vi "HEWH RLT Gather Serial Data.vi"(0 "Serial Port Ref":refnum<visa-resource-name>="COM3", 5 "GEA2 HyperData":bool, 11 "error in (no error)":errorcluster) -> (4 "Serial Data B":string[][](array[string]), 15 "error out":errorcluster)   [LabVIEW 2014]
uses:
  Support VIs/Global HEWH.vi
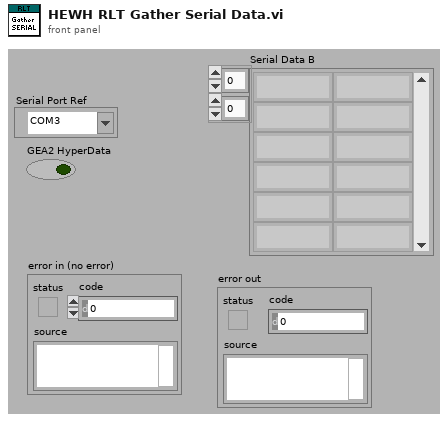
[diagram p1: front panel]
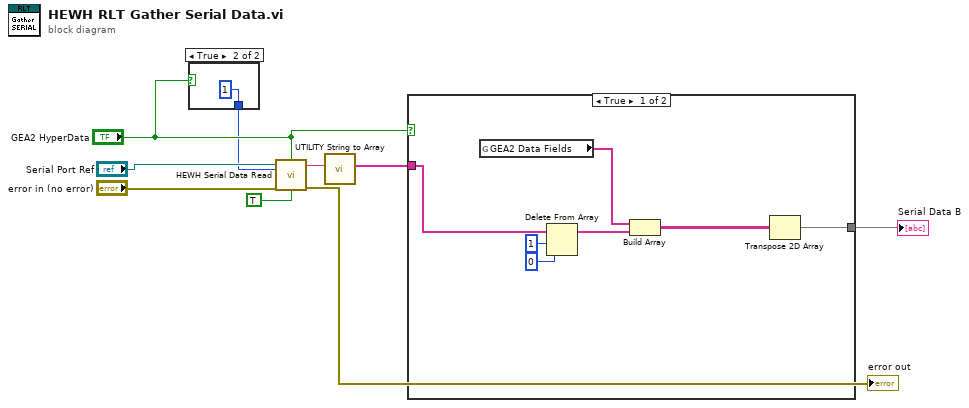
[diagram p0: block diagram]
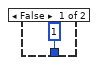
[diagram p2: hidden frame]
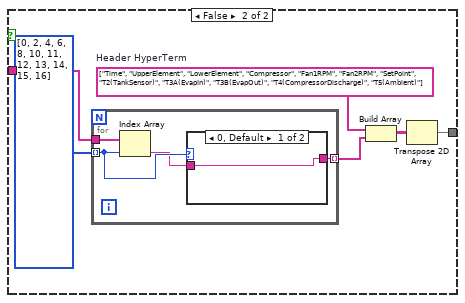
[diagram p3: hidden frame]
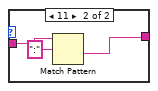
[diagram p4: hidden frame]
diagram:
  n1 = case shown="True" "GEA2 HyperData" {
    tunnel: [1 ("Retries") 1 ("Retries")] -> w1
    frame False {
    }
    frame True {
    }
  }
  n2 = call "HEWH Serial Data Read.vi"("Serial Port Ref"="Serial Port Ref", "GEA2 HyperData"="GEA2 HyperData", "Retries"=w1, "error in (no error)"="error in (no error)", "Enable Clear Buf."=TRUE) -> ("Read String"=w6:string, "error out"=→"error out":errorcluster)  [unwired: 7 in, 2 out]
  n3 = call "UTILITY String to Array.vi"("String"=w6) -> ("Array"=w7:string[])  [unwired: 10 in]
  n4 = case shown="True" "GEA2 HyperData" {
    tunnel: w7 -> [w14 w23]
    tunnel: [w17 w19] -> w5
    frame True {
      n5 = global read "Global HEWH.vi" "GEA2 Data Fields"() -> (w16:string[])
      n6 = Delete From Array(array=w14, length=1, index=0) -> (array with subset deleted=w15:string[])  [unwired: 1 out]
      n7 = Build Array(w16, w15) -> (w18:string[][])
      n8 = Transpose 2D Array(2D array=w18) -> (transposed array=w17:string[][])
    }
    frame False {
      w22 = string[] ["Time", "UpperElement", "LowerElement", "Compressor", "Fan1RPM", "Fan2RPM", "SetPoint", "T2(TankSensor)", "T3A(EvapIn)", "T3B(EvapOut)", "T4(CompressorDischarge)", "T5(Ambient)"]  # Header HyperTerm
      n9 = for {
        tunnel: w23 -> [w28]
        tunnel: i32[] [0, 2, 4, 6, 8, 10, 11, 12, 13, 14, 15, 16] -> [w27] mode=indexing
        tunnel: [w25] -> w21 mode=indexing
        n10 = Index Array(array=w28, index=w27) -> (element=w26:string)
        n11 = case shown="0, Default" w27 {
          tunnel: w26 -> [w29 w32]
          tunnel: [w29 w30] -> w25
          frame 0, Default {
          }
          frame 11 {
            n12 = Match Pattern(string=w32, regular expression=":") -> (after substring=w30:string)  [unwired: 1 in, 3 out]
          }
        }
      }
      n13 = Build Array(w22, w21) -> (w20:string[][])
      n14 = Transpose 2D Array(2D array=w20) -> (transposed array=w19:string[][])
    }
  }
  "Serial Data B" <- w5
